vi "Update.vi"(8 "error in (no error)":errorcluster, 10 "Text":string, 11 "Normal Text in":refnum<class "Normal Text.lvclass">) -> (0 "error out":errorcluster, 3 "Normal Text out":refnum<class "Normal Text.lvclass">)   [LabVIEW 2011, in "Normal Text.lvclass"]
uses:
  Normal Text.lvclass
  Normal Text.lvclass/Normal Text.ctl
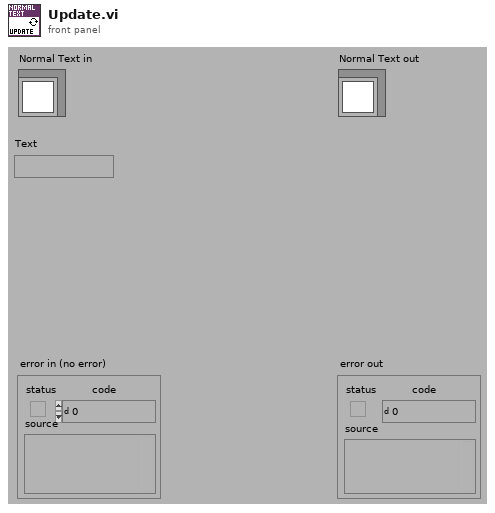
[diagram p1: front panel]
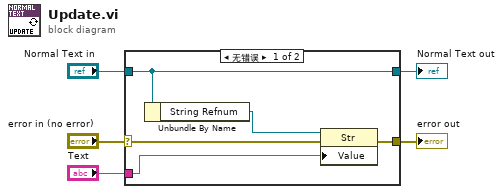
[diagram p0: block diagram]
diagram:
  n1 = case shown="无错误" "error in (no error)" {
    selector: "error in (no error)" -> [w8 w12]
    tunnel: "Normal Text in" -> [w6 w11]
    tunnel: "Text" -> [w9 _]
    tunnel: [w7 w12] -> w2
    tunnel: [w6 w11] -> w1
    frame No Error {
      n2 = Unbundle By Name(w6) -> ("String Refnum"=w10:refnum<vi>)
      n3 = property class="Str"(reference=w10, error in=w8, "Value"=w9) -> (error out=w7:errorcluster)  [unwired: 1 out]
    }
    frame Error {
    }
  }
  "Normal Text out" <- w1
  "error out" <- w2
